vi "$OLS_LevelZeroVerification.vi"() -> ()   [LabVIEW 2024]
doc: "Used to verify and calculate the Level Zero offset value. The User is Prompted for their NAME, then the Level is set to 5 evaluation Set Points (SP). Onece the SP is reached the User should measure the oil level from the datum then recored the MEASURED Level in Inches when prompted. Once all five measuremnts are complete, the results are fit using LSR, a residual plot is displayed and the user is prompted to select an Excel workbook to which the results are appended on sheet 1. \n\nUse the STOP button to interrupt and end the Zero process."
uses:
  Control Definitions/Def_CalState_Enum.ctl
  Control Definitions/Def_PumpSpeed.ctl
  Control Definitions/DEF_PumpManCtl.ctl
  Control Definitions/DEF_PumpParams.ctl
  <vilib>/Analysis/NI_AALPro.lvlib
panel:
  out "Constant":dbl format="%.4g"
  out "Auto/!Man":bool=TRUE
  in  "Pump Params":T1={"Empty Inches"=1.1, "Full Inches"=7.2, "RNG_SLOW"=0.5, "RNG_CREEP"=0.007, "RNG_STOP "=0.002, "VISA resource name"="COM4", "SPD_SLOW"=30, "SPD_CREEP"=10, "SPD_FAST"=100, "Zero template"=path "C:/AllenProjects/PWC-OLS/$Calibrtation/CAL_Level_RnR_241105.xlsx", "zero  Settle sec"=5.0} {"RNG_STOP" format="%#_13g"; "RNG_CREEP" format="%#_13g"; "RNG_SLOW" format="%#_13g"}
  in  "Pump Manual Controls":T2={"Pump Speed"=enum."STOP", "FILL"=FALSE, "Drain"=FALSE, "Auto/!Man"=TRUE, "Sim Level"=FALSE}
  out "Msg":string
  out "Pump Status":bool=TRUE
  out "Residual Plot":dbl[](graph)=[-0.0, -0.0, -0.0, -0.0, -0.0]
  out "Offest":dbl=-0.0 format="%.4g"
  out "Slope":dbl=-0.0 format="%.4g"
  out "Time":string="11/17/2024 3:56 PM"
  out "Name":string="rob"
  in  "Stop Pump":bool=TRUE
  out "Calibration":cluster{"SP":dbl, "Laser":dbl, "Measure":dbl}[](array[cluster])=[{"SP"=1.1, "Laser"=1.102, "Measure"=0.0}, {"SP"=2.7229265223579855, "Laser"=2.7239999999999855, "Measure"=0.0}, {"SP"=4.174679755518124, "Laser"=4.173999999999982, "Measure"=0.0}, {"SP"=5.682906773962424, "Laser"=5.6819999999999755, "Measure"=0.0}, {"SP"=7.199999999999999, "Laser"=7.203999999999969, "Measure"=0.0}] {"Measure" format="%.3g"; "Laser" format="%.3g"; "SP" format="%.3g"}
  out "Count":i32=5
  out "Pump Speed Out":T3=enum."CREEP"
  out "State Var":T4=enum."Done"
  in  "stop":bool
  out "Level PV":dbl(slide)=7.203999999999969 scale=0.0..10.0
  in  "Level SP":dbl(slide)=7.199999999999999 scale=0.0..10.0
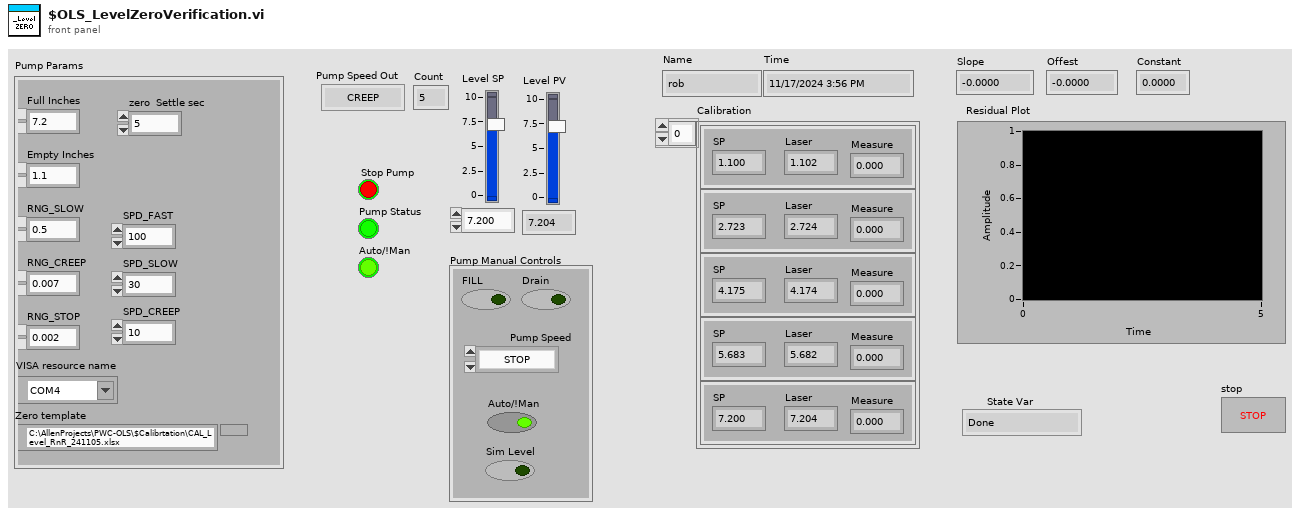
[diagram p1: front panel]
types:
  T1 = typedef "DEF_PumpParams.ctl" = cluster{"Empty Inches":dbl, "Full Inches":dbl, "RNG_SLOW":dbl, "RNG_CREEP":dbl, "RNG_STOP ":dbl, "VISA resource name":refnum<visa-resource-name>, "SPD_SLOW":i32, "SPD_CREEP":i32, "SPD_FAST":i32, "Zero template":path, "zero  Settle sec":dbl}
  T2 = typedef "DEF_PumpManCtl.ctl" = cluster{"Pump Speed":T3, "FILL":bool, "Drain":bool, "Auto/!Man":bool, "Sim Level":bool}
  T3 = typedef "Def_PumpSpeed.ctl" = enum16{"FAST", "SLOW", "CREEP", "STOP"}
  T4 = typedef "Def_CalState_Enum.ctl" = enum16{"Start", "Get Info", "Get SP", "Going to SP", "Wait Settle", "Get Measure", "Save Measure", "Done", "Manual"}
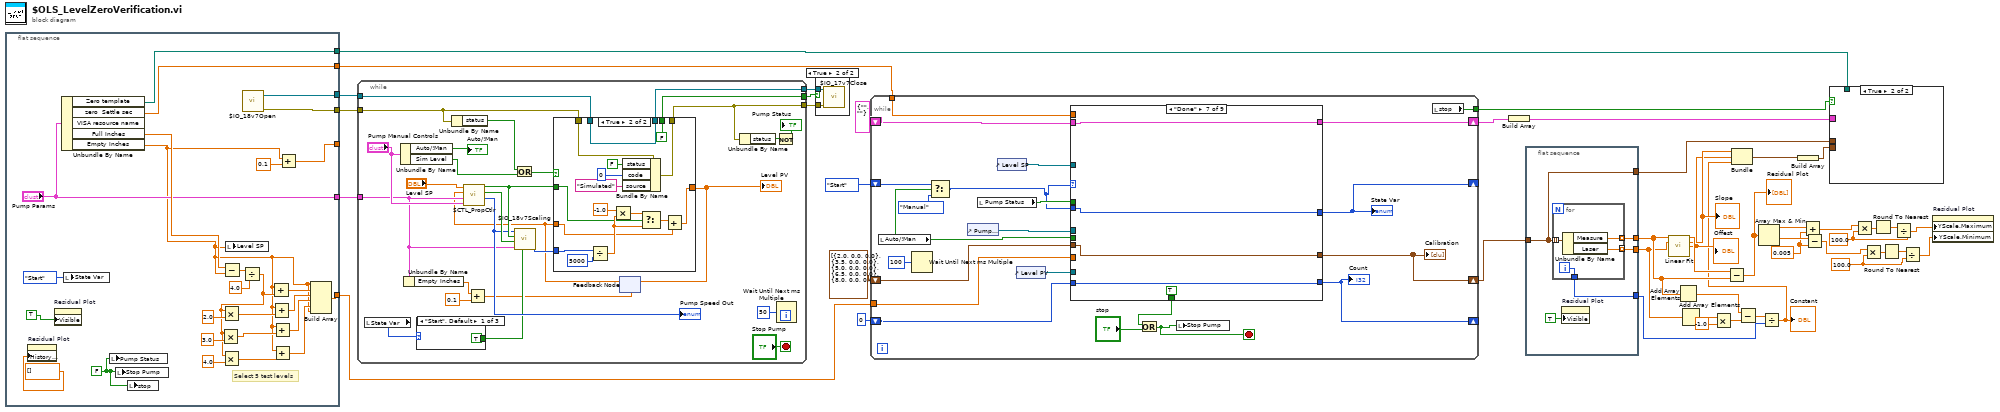
[diagram p0: block diagram]
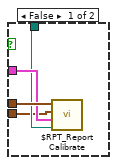
[diagram p3: hidden frame]
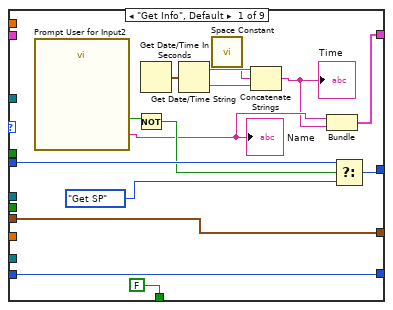
[diagram p4: hidden frame]
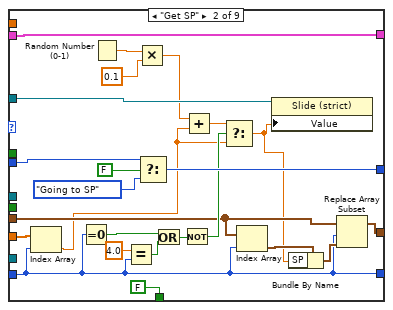
[diagram p5: hidden frame]
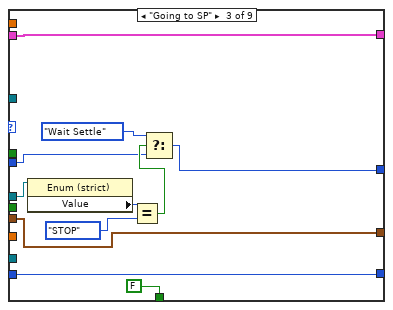
[diagram p6: hidden frame]
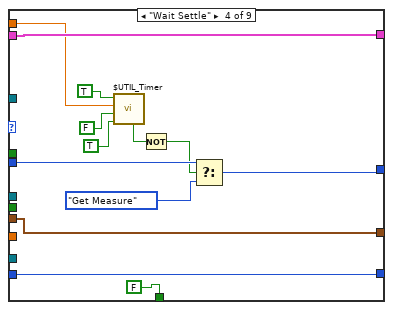
[diagram p7: hidden frame]
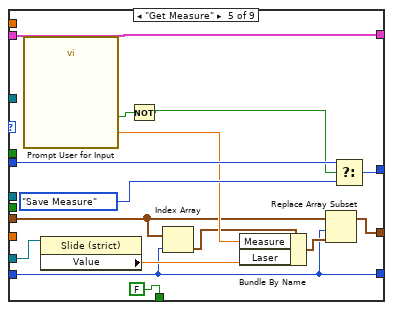
[diagram p8: hidden frame]
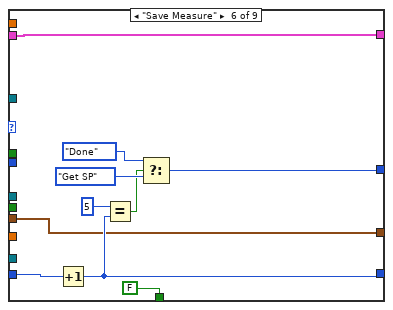
[diagram p9: hidden frame]
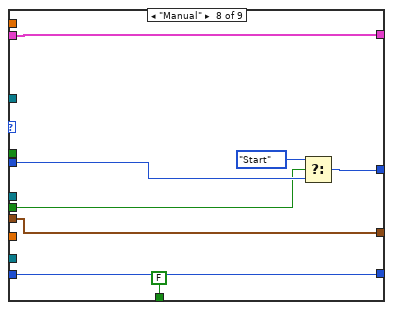
[diagram p10: hidden frame]
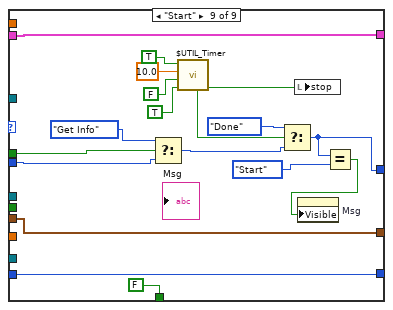
[diagram p11: hidden frame]
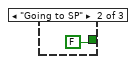
[diagram p12: hidden frame]
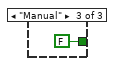
[diagram p13: hidden frame]
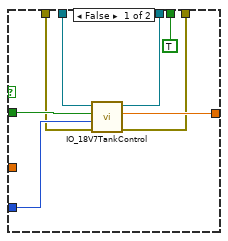
[diagram p14: hidden frame]
diagram:
  w18 = 100.0 ("y")
  w25 = 100.0 ("y")
  w41 = 0.005 ("y")
  n1 = flat-sequence {
    tunnel: [w49] -> _
    tunnel: [w59] -> w33
    tunnel: [w57] -> w30
    tunnel: [w56] -> w29
    tunnel: ["Pump Params"] -> w17
    tunnel: [w48] -> w13
    tunnel: [w47] -> w12
    frame #0 {
      w55 = FALSE
      # "Select 5 test levels"
      n2 = property on="Residual Plot" class="WFChart (strict)"("History Data"=dbl[] []) -> ()  [unwired: 2 in, 2 out]
      n3 = property on="Residual Plot" class="WFChart (strict)"("Visible"=TRUE) -> ()  [unwired: 2 in, 2 out]
      n4 = Unbundle By Name("Pump Params") -> ("Zero template"=w48:path, "zero  Settle sec"=w47:dbl, "Full Inches"=w54:dbl, "Empty Inches"=w50:dbl)  [unwired: 1 out]
      n5 = local write "State Var"(Def_CalState_Enum."Start" ("State Var")) -> ()
      n6 = local write "Pump Status"(w55) -> ()
      n7 = local write "Stop Pump"(w55) -> ()
      n8 = local write "stop"(w55) -> ()
      n9 = Subtract(x=w54, y=w50) -> (x-y=w71:dbl)
      n10 = local write "Level SP"(w50) -> ()
      n11 = Divide(x=w71, y=4.0) -> (x/y=w58:dbl)
      n12 = Multiply(x=w58, y=3.0) -> (x*y=w64:dbl)
      n13 = Multiply(x=w58, y=2.0) -> (x*y=w67:dbl)
      n14 = Multiply(x=w58, y=4.0) -> (x*y=w63:dbl)
      n15 = call "$IO_18v7Open.vi"() -> ("error out"=w56:errorcluster, "VISA Refnum out"=w57:refnum<visa-resource-name>)  [unwired: 10 in]
      n16 = Add(x=w50, y=w58) -> (x+y=w68:dbl)
      n17 = Add(x=w50, y=w67) -> (x+y=w62:dbl)
      n18 = Add(x=w50, y=w64) -> (x+y=w61:dbl)
      n19 = Add(x=w50, y=w63) -> (x+y=w60:dbl)
      n20 = Add(x=w50, y=0.1) -> (x+y=w49:dbl)
      n21 = Build Array(w50, w68, w62, w61, w60, w50) -> (w59:dbl[])
    }
  }
  n22 = while {
    tunnel: [w97] -> w32
    tunnel: [w91] -> w31
    tunnel: w30 -> [w96]
    tunnel: w29 -> [w77]
    tunnel: w17 -> [w82]
    tunnel: [w86] -> w16
    stop <- "Stop Pump" stop-if-true
    n23 = local read "State Var"() -> (w88:T4)
    n24 = Unbundle By Name("Pump Manual Controls") -> ("Auto/!Man"=→"Auto/!Man":bool, "Sim Level"=w75:bool)
    n25 = Unbundle By Name(w82) -> ("Empty Inches"=w81:dbl)
    n26 = case shown="\"Start\", Default" w88 {
      tunnel: [TRUE FALSE FALSE] -> w87
      frame "Start", Default {
      }
      frame "Going to SP" {
      }
      frame "Manual" {
      }
    }
    n27 = Unbundle By Name(w77) -> ("status"=w74:bool)
    n28 = Add(x=w81, y=0.1) -> (x+y=w78:dbl)
    n29 = Or(x=w74, y=w75) -> (x .or. y?=w76:bool)
    n30 = feedback #1(w78) -> (w79:dbl)
    n31 = call "$CTL_PropCtlr.vi"("Pump Manual Controls"="Pump Manual Controls", "Pump Params"=w82, "Level PV"=w79, "Level SP"="Level SP") -> ("Pump Speed Out"=w93:T3, "X< Neg"=w95:bool, "X>Pos"=w94:bool)  [unwired: 4 in, 1 out]
    "Pump Speed Out" <- w93
    n32 = call "$IO_18v7Scaling.vi"("!Enabled"=w87, "Pump Params"=w82, "Drain"=w95, "Fill"=w94, "Pump Speed"=w93) -> ("Speed Out"=w92:i32)  [unwired: 5 in, 1 out]
    n33 = case shown="True" w76 {
      tunnel: w79 -> [_ w117]
      tunnel: [w111 w118] -> w80
      tunnel: w94 -> [w110 w119]
      tunnel: w92 -> [w109 w122]
      tunnel: [w108 w123] -> w97
      tunnel: [w107 w112] -> w91
      tunnel: w96 -> [w106 w123]
      tunnel: w77 -> [w105 w116]
      tunnel: [TRUE FALSE] -> w86
      frame False {
        n34 = call "IO_18V7TankControl.vi"("error in"=w105, "Speed"=w109, "Fill!Drain"=w110, "VISA Refnum in"=w106) -> ("error out"=w107:errorcluster, "Laser Raw"=w111:sgl, "VISA Refnum out"=w108:refnum<visa-resource-name>)  [unwired: 4 in, 1 out]
      }
      frame True {
        n35 = Divide(x=w122, y=5000) -> (x/y=w125:dbl)
        n36 = Multiply(x=-1.0 ("y"), y=w125) -> (x*y=w126:dbl)
        n37 = Bundle By Name(cluster=w116, "status"=FALSE, "code"=0, "source"="Simulated") -> (w112:errorcluster)
        n38 = Select(t=w126, s=w119, f=w125) -> (s? t:f=w121:dbl)
        n39 = Add(x=w121, y=w117) -> (x+y=w118:dbl)
      }
    }
    "Level PV" <- w80
    n40 = feedback-in #1(w80) -> ()
    n41 = Unbundle By Name(w91) -> ("status"=w90:bool)
    n42 = Not(x=w90) -> (.not. x?=→"Pump Status":bool)
    n43 = Wait Until Next ms Multiple(millisecond multiple=u32 50) -> ()  [unwired: 1 out]
  }
  n44 = case shown="True" w16 {
    tunnel: w32 -> [_ w129]
    tunnel: w31 -> [_ w128]
    frame False {
    }
    frame True {
      n45 = call "$IO_17v7Close.vi"("error in (no error)"=w128, "VISA Refnum in"=w129) -> ()  [unwired: 10 in]
    }
  }
  n46 = while {
    shift-right: [w150] -> _
    shift-left: Def_CalState_Enum."Start" ("f") -> [w134]
    shift-right: [w143] -> _
    shift-left: 0 -> [w146]
    shift-right: [w141] -> w14
    shift-left: cluster{"SP":dbl, "Laser":dbl, "Measure":dbl}[] [{"SP"=2.0, "Laser"=0.0, "Measure"=0.0}, {"SP"=3.5, "Laser"=0.0, "Measure"=0.0}, {"SP"=5.0, "Laser"=0.0, "Measure"=0.0}, {"SP"=6.5, "Laser"=0.0, "Measure"=0.0}, {"SP"=8.0, "Laser"=0.0, "Measure"=0.0}] ("Calibration") -> [w142]
    shift-right: [w140] -> w36
    shift-left: cluster{"Name":string, string} {"Name"="", ""} -> [w139]
    tunnel: w33 -> [w138]
    tunnel: [w136] -> w28
    tunnel: w12 -> [w130]
    stop <- w145 stop-if-true
    n47 = local read "Auto/!Man"() -> (w131:bool)
    n48 = Wait Until Next ms Multiple(millisecond multiple=u32 100) -> ()  [unwired: 1 out]
    n49 = Select(t=w134, s=w131, f=Def_CalState_Enum."Manual") -> (s? t:f=w133:T4)
    n50 = control-ref of="Pump Speed Out"() -> (w149:refnum<vi>)
    n51 = local read "Pump Status"() -> (w135:bool)
    n52 = control-ref of="Level SP"() -> (w147:refnum<vi>)
    n53 = control-ref of="Level PV"() -> (w144:refnum<vi>)
    n54 = case shown="\"Done\"" w133 {
      tunnel: [w164 w188 w201 w203 w229 w232 w244 w249 w255] -> w150
      tunnel: w133 -> [w165 w189 w197 w213 w228 _ w244 w248 w267]
      tunnel: w149 -> [_ _ w196 _ _ _ _ _ _]
      tunnel: w146 -> [w163 w168 w194 w212 w216 w239 w243 w250 w269]
      tunnel: [w163 w168 w194 w212 w216 w238 w243 w250 w269] -> w143
      tunnel: [FALSE FALSE FALSE FALSE FALSE FALSE TRUE FALSE FALSE] -> w148
      tunnel: w147 -> [_ w186 _ _ _ _ _ _ _]
      tunnel: w144 -> [_ _ _ _ w220 _ _ _ _]
      tunnel: w142 -> [w161 w172 w192 w205 w217 w231 w241 w251 w270]
      tunnel: [w161 w171 w192 w205 w221 w231 w241 w251 w270] -> w141
      tunnel: [w154 w184 w191 w204 w218 w230 w240 w252 w268] -> w140
      tunnel: w139 -> [_ w184 w191 w204 w218 w230 w240 w252 w268]
      tunnel: w138 -> [_ w174 _ _ _ _ _ _ _]
      tunnel: w135 -> [_ _ _ _ _ _ _ _ w266]
      tunnel: w131 -> [_ _ _ _ _ _ _ w246 _]
      tunnel: w130 -> [_ _ _ w202 _ _ _ _ _]
      frame "Get Info", Default {
        n55 = call "Prompt User for Input2"() -> ("Name"=w156:string, "OK"=w160:bool)  [unwired: 17 in, 1 out]
        "Name" <- w156
        n56 = Not(x=w160) -> (.not. x?=w159:bool)
        n57 = Get Date/Time In Seconds() -> (seconds since 1Jan1904=w158:timestamp)
        n58 = Get Date/Time String(seconds (now)=w158) -> (date string=w157:string, time string=w153:string)  [unwired: 2 in]
        n59 = call <vilib>:"Space Constant.vi"() -> ("String"=w152:string)
        n60 = Concatenate Strings(w157, w152, w153) -> (w155:string)
        "Time" <- w155
        n61 = Bundle("Name"=w156, w155) -> (w154:cluster{"Name":string, string})  [unwired: 1 in]
        n62 = Select(t=w165, s=w159, f=Def_CalState_Enum."Get SP") -> (s? t:f=w164:T4)
      }
      frame "Get SP" {
        n63 = Index Array(array=w174, index=w168) -> (element=w170:dbl)
        n64 = Equal To 0?(x=w168) -> (x = 0?=w178:bool)
        n65 = Random Number (0-1)() -> (number: 0 to 1=w182:dbl)
        n66 = Equal?(x=4.0 ("y"), y=w168) -> (x = y?=w179:bool)
        n67 = Multiply(x=w182, y=0.1) -> (x*y=w181:dbl)
        n68 = Select(t=w189, s=FALSE ("s 2"), f=Def_CalState_Enum."Going to SP") -> (s? t:f=w188:T4)
        n69 = Or(x=w178, y=w179) -> (x .or. y?=w177:bool)
        n70 = Not(x=w177) -> (.not. x?=w176:bool)
        n71 = Add(x=w181, y=w170) -> (x+y=w175:dbl)
        n72 = Select(t=w175, s=w176, f=w170) -> (s? t:f=w167:dbl)
        n73 = Index Array(array=w172, index=w168) -> (element=w173:cluster{"SP":dbl, "Laser":dbl, "Measure":dbl})
        n74 = property class="Slide (strict)"(reference=w186, "Value"=w167) -> ()  [unwired: 1 in, 2 out]
        n75 = Bundle By Name(cluster=w173, "SP"=w167) -> (w169:cluster{"SP":dbl, "Laser":dbl, "Measure":dbl})
        n76 = Replace Array Subset(array=w172, new element=w169, index=w168) -> (w171:cluster{"SP":dbl, "Laser":dbl, "Measure":dbl}[])
      }
      frame "Going to SP" {
        n77 = property class="Enum (strict)"(reference=w196) -> ("Value"=w195:T3)  [unwired: 1 in, 2 out]
        n78 = Equal?(x=w195, y=Def_PumpSpeed."STOP") -> (x = y?=w200:bool)
        n79 = Select(t=Def_CalState_Enum."Wait Settle" ("f"), s=w200, f=w197) -> (s? t:f=w201:T4)
      }
      frame "Wait Settle" {
        n80 = call "$UTIL_Timer.vi"("Auto Reset"=TRUE, "Reset"=FALSE, "Time (sec)"=w202, "Start"=TRUE) -> ("TO Trig"=w208:bool)  [unwired: 2 in, 5 out]
        n81 = Not(x=w208) -> (.not. x?=w207:bool)
        n82 = Select(t=w213, s=w207, f=Def_CalState_Enum."Get Measure") -> (s? t:f=w203:T4)
      }
      frame "Get Measure" {
        n83 = call "Prompt User for Input"() -> ("Measure"=w225:dbl, "OK"=w224:bool)  [unwired: 17 in, 1 out]
        n84 = property class="Slide (strict)"(reference=w220) -> ("Value"=w219:dbl)  [unwired: 1 in, 2 out]
        n85 = Not(x=w224) -> (.not. x?=w223:bool)
        n86 = Index Array(array=w217, index=w216) -> (element=w215:cluster{"SP":dbl, "Laser":dbl, "Measure":dbl})
        n87 = Bundle By Name(cluster=w215, "Measure"=w225, "Laser"=w219) -> (w222:cluster{"SP":dbl, "Laser":dbl, "Measure":dbl})
        n88 = Replace Array Subset(array=w217, new element=w222, index=w216) -> (w221:cluster{"SP":dbl, "Laser":dbl, "Measure":dbl}[])
        n89 = Select(t=w228, s=w223, f=Def_CalState_Enum."Save Measure") -> (s? t:f=w229:T4)
      }
      frame "Save Measure" {
        n90 = Increment(x=w239) -> (x+1=w238:i32)
        n91 = Equal?(x=5, y=w238) -> (x = y?=w234:bool)
        n92 = Select(t=Def_CalState_Enum."Done" ("f"), s=w234, f=Def_CalState_Enum."Get SP") -> (s? t:f=w232:T4)
      }
      frame "Done" {
      }
      frame "Manual" {
        n93 = Select(t=Def_CalState_Enum."Start", s=w246, f=w248) -> (s? t:f=w249:T4)
      }
      frame "Start" {
        n94 = Select(t=Def_CalState_Enum."Get Info", s=w266, f=w267) -> (s? t:f=w258:T4)
        n95 = call "$UTIL_Timer.vi"("Auto Reset"=TRUE, "Reset"=FALSE, "Time (sec)"=10.0, "Start"=TRUE) -> ("Timed Out"=w256:bool, "TO Trig"=w257:bool)  [unwired: 2 in, 4 out]
        n96 = Select(t=Def_CalState_Enum."Done", s=w257, f=w258) -> (s? t:f=w255:T4)
        n97 = local write "stop"(w256) -> ()
        n98 = Equal?(x=w255, y=Def_CalState_Enum."Start" ("t")) -> (x = y?=w253:bool)
        n99 = property on="Msg" class="Str"("Visible"=w253) -> ()  [unwired: 2 in, 2 out]
      }
    }
    "State Var" <- w150
    "Count" <- w143
    "Calibration" <- w141
    n100 = Or(x=w148, y="stop") -> (x .or. y?=w145:bool)
    n101 = local write "Stop Pump"(w145) -> ()
    n102 = local read "stop"() -> (w136:bool)
  }
  n103 = Build Array(w36) -> (w35:cluster{"Name":string, string}[])
  n104 = flat-sequence {
    tunnel: [w275] -> w11
    tunnel: [w274] -> w10
    tunnel: w14 -> [w272]
    tunnel: [w272] -> w15
    tunnel: [w271] -> w4
    frame #0 {
      n105 = for {
        tunnel: w272 -> [w279] mode=indexing
        tunnel: [w278] -> w275 mode=indexing
        tunnel: [w277] -> w274 mode=indexing
        tunnel: [w276] -> w271
        i -> [w276]
        n106 = Unbundle By Name(w279) -> ("Measure"=w278:dbl, "Laser"=w277:dbl)
      }
      n107 = property on="Residual Plot" class="WFChart (strict)"("Visible"=TRUE) -> ()  [unwired: 2 in, 2 out]
    }
  }
  n108 = call <vilib>:"Linear Fit.vi"("Y"=w11, "X"=w10) -> ("Best Linear Fit"=w44:dbl[], "slope"=w39:dbl, "intercept"=w38:dbl)  [unwired: 9 in, 2 out]
  "Slope" <- w39
  "Offest" <- w38
  n109 = Add Array Elements(numeric array=w11) -> (sum=w6:dbl)
  n110 = Add Array Elements(numeric array=w10) -> (sum=w9:dbl)
  n111 = Multiply(x=w9, y=-1.0) -> (x*y=w7:dbl)
  n112 = Subtract(x=w44, y=w11) -> (x-y=w43:dbl[])
  "Residual Plot" <- w43
  n113 = Subtract(x=w6, y=w7) -> (x-y=w5:dbl)
  n114 = Array Max & Min(array=w43) -> (max value=w40:dbl, min value=w42:dbl)  [unwired: 2 out]
  n115 = Divide(x=w5, y=w4) -> (x/y=w3:dbl)
  "Constant" <- w3
  n116 = Bundle("slope"=w39, "intercept"=w38, w3) -> (w2:cluster{"slope":dbl, "intercept":dbl, dbl})  [unwired: 1 in]
  n117 = Build Array(w2) -> (w1:cluster{"slope":dbl, "intercept":dbl, dbl}[])
  n118 = Add(x=w40, y=w41) -> (x+y=w24:dbl)
  n119 = Subtract(x=w42, y=w41) -> (x-y=w19:dbl)
  n120 = case shown="True" w28 {
    tunnel: w15 -> [w283 _]
    tunnel: w35 -> [w282 _]
    tunnel: w13 -> [w281 _]
    tunnel: w1 -> [w280 _]
    frame False {
      n121 = call "$RPT_Report Calibrate.vi"("template"=w281, "Info"=w282, "LinEq"=w280, "Calibration"=w283) -> ()  [unwired: 8 in]
    }
    frame True {
    }
  }
  n122 = Multiply(x=w24, y=w25) -> (x*y=w26:dbl)
  n123 = Multiply(x=w19, y=w18) -> (x*y=w21:dbl)
  n124 = Round To Nearest(number=w26) -> (nearest integer value=w27:dbl)
  n125 = Round To Nearest(number=w21) -> (nearest integer value=w22:dbl)
  n126 = Divide(x=w27, y=w25) -> (x/y=w23:dbl)
  n127 = Divide(x=w22, y=w18) -> (x/y=w20:dbl)
  n128 = property on="Residual Plot" class="WFChart (strict)"("YScale.Maximum"=w23, "YScale.Minimum"=w20) -> ()  [unwired: 2 in, 2 out]
